vi "Configure Control Loop Response Power Analysis (Frequency).vi"(6 "Stop Frequency (6: 20000000 Hz)":i32(ring)=6 items=["100", "1000", "10000", "100000", "1000000", "10000000", "20000000"], 7 "Single Frequency (1: 100 Hz)":i32(ring)=1 items=["20", "100", "1000", "10000", "100000", "1000000", "10000000", "2000000"], 8 "error in (no error)":errorcluster, 9 "Start Frequency (1: 100 Hz)":i32(ring)=1 items=["20", "100", "1000", "10000", "100000", "1000000", "10000000"], 10 "Frequency Mode (0: Sweep)":i32(ring) items=["Sweep", "Single"], 11 "VISA resource name":refnum<visa-resource-name>) -> (0 "error out":errorcluster, 3 "VISA resource name out":refnum<visa-resource-name>)   [LabVIEW 2017, in "Agilent 2000 3000 X-Series.lvlib"]
doc: "Configures the frequency for control loop response power analysis.\n\n<b>Note:</b>\n - This VI is applicable for 3000T, 3000G, 4000, 6000 X-Series."
uses:
  Agilent 2000 3000 X-Series.lvlib
panel:
  # "Single Mode"
  # "Sweep Mode"
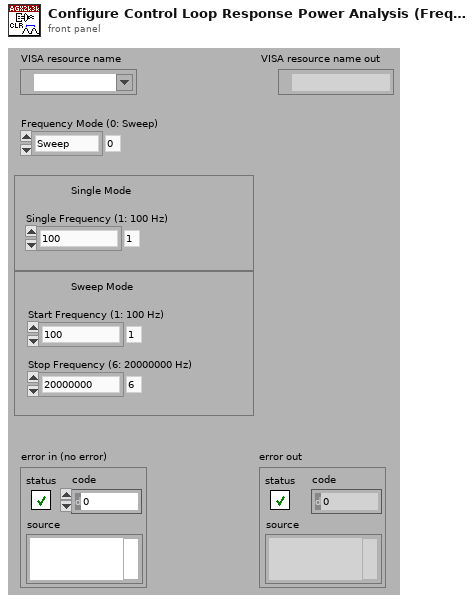
[diagram p1: front panel]
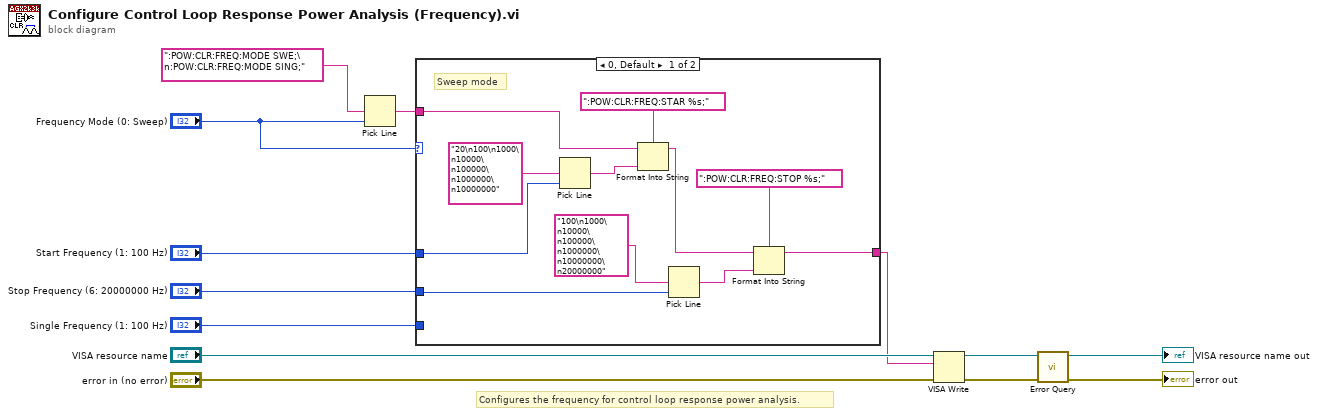
[diagram p0: block diagram]
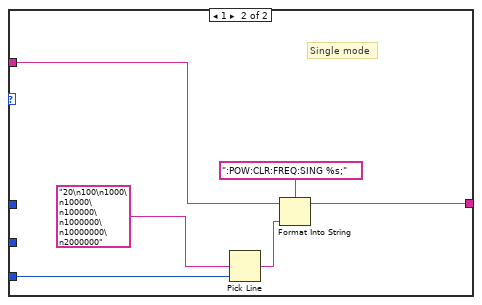
[diagram p2: hidden frame]
diagram:
  # "Configures the frequency for control loop response power analysis."
  n1 = Pick Line(multi-line string=":POW:CLR:FREQ:MODE SWE;\n:POW:CLR:FREQ:MODE SING;", line index="Frequency Mode (0: Sweep)") -> (output string=w4:string)  [unwired: 1 in]
  n2 = case shown="0, Default" "Frequency Mode (0: Sweep)" {
    tunnel: "Single Frequency (1: 100 Hz)" -> [_ w26]
    tunnel: w4 -> [w21 w29]
    tunnel: [w15 w28] -> w3
    tunnel: "Start Frequency (1: 100 Hz)" -> [w20 _]
    tunnel: "Stop Frequency (6: 20000000 Hz)" -> [w19 _]
    frame 0, Default {
      # "Sweep mode"
      n3 = Pick Line(multi-line string="20\n100\n1000\n10000\n100000\n1000000\n10000000", line index=w20) -> (output string=w23:string)  [unwired: 1 in]
      n4 = Format Into String(format string=":POW:CLR:FREQ:STAR %s;", initial string=w21, w23) -> (resulting string=w14:string)  [unwired: 1 in, 1 out]
      n5 = Pick Line(multi-line string="100\n1000\n10000\n100000\n1000000\n10000000\n20000000", line index=w19) -> (output string=w17:string)  [unwired: 1 in]
      n6 = Format Into String(format string=":POW:CLR:FREQ:STOP %s;", initial string=w14, w17) -> (resulting string=w15:string)  [unwired: 1 in, 1 out]
    }
    frame 1 {
      # "Single mode"
      n7 = Pick Line(multi-line string="20\n100\n1000\n10000\n100000\n1000000\n10000000\n2000000", line index=w26) -> (output string=w27:string)  [unwired: 1 in]
      n8 = Format Into String(format string=":POW:CLR:FREQ:SING %s;", initial string=w29, w27) -> (resulting string=w28:string)  [unwired: 1 in, 1 out]
    }
  }
  n9 = VISA Write(VISA resource name="VISA resource name", write buffer=w3, error in (no error)="error in (no error)") -> (VISA resource name out=w10:refnum<visa-resource-name>, error out=w9:errorcluster)  [unwired: 1 out]
  n10 = call "Error Query.vi"("error in (no error)"=w9, "VISA resource name"=w10) -> ("error out"=→"error out":errorcluster, "VISA resource name out"=→"VISA resource name out":refnum<visa-resource-name>)  [unwired: 6 in, 2 out]
